vi "format_frame.vi"(6 "mask?":bool, 7 "hangup status code":T1 items=["ignore"=0, "normal"=1000, "going away"=1001, "protocol error"=1002, "invalid data"=1003], 9 "fin?":bool, 10 "data in":string, 11 "opcode":T2 items=["continue"=0, "text"=1, "binary"=2, "hangup"=8, "ping"=9, "pong"=10]) -> (3 "frame data out":string)   [LabVIEW 2019, in "WebSocket Server Toolkit.lvlib"]
uses:
  WebSocket Server Toolkit.lvlib
  types/opcode.ctl
  types/status_code.ctl
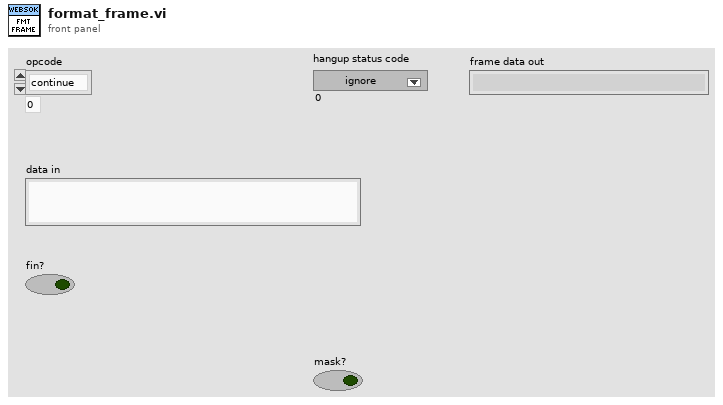
[diagram p1: front panel]
types:
  T1 = typedef "WebSocket Server Toolkit.lvlib/status_code.ctl" = u16
  T2 = typedef "WebSocket Server Toolkit.lvlib/opcode.ctl" = u8
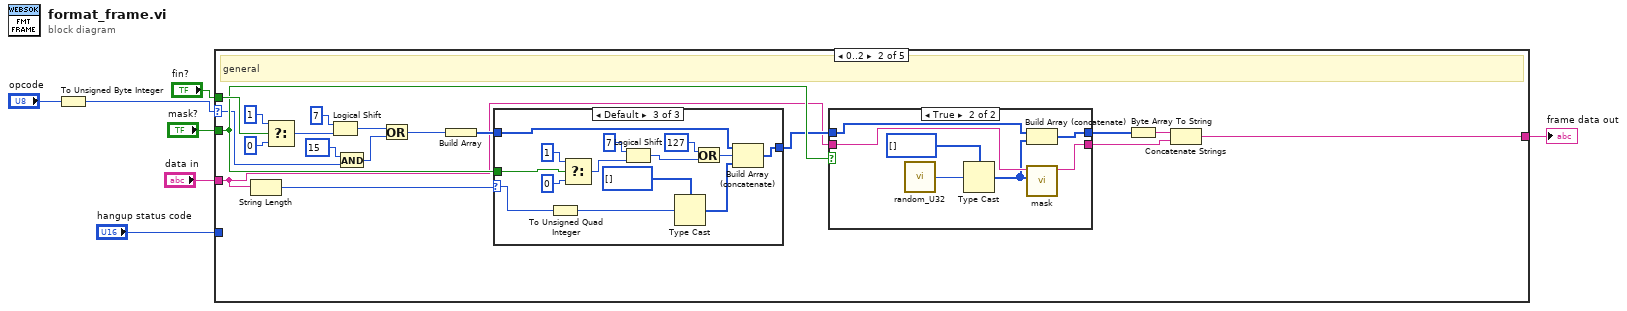
[diagram p0: block diagram]
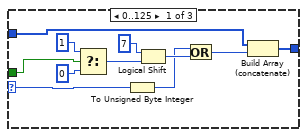
[diagram p4: hidden frame]
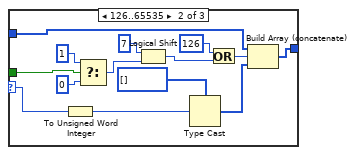
[diagram p5: hidden frame]
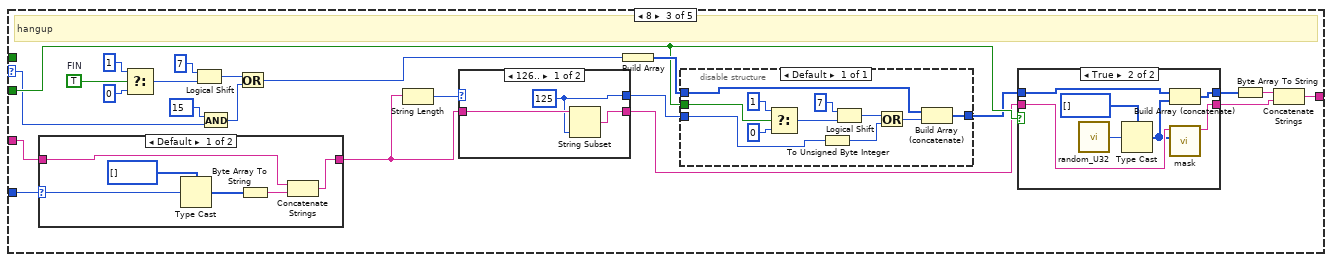
[diagram p6: hidden frame]
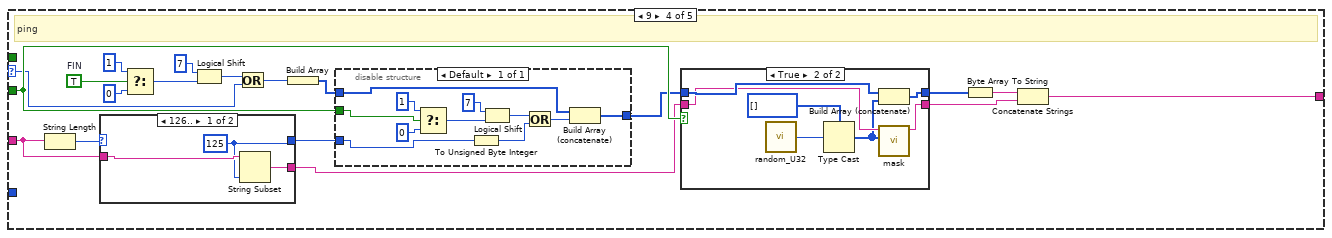
[diagram p10: hidden frame]
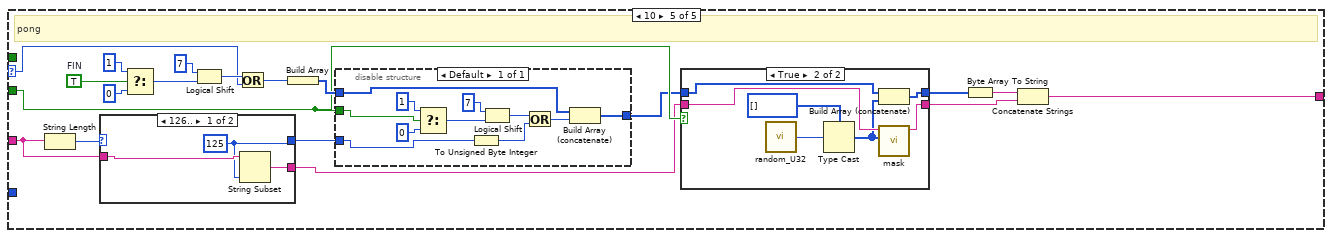
[diagram p13: hidden frame]
diagram:
  n1 = To Unsigned Byte Integer(number="opcode") -> (unsigned 8bit integer=w3:T2)
  n2 = case shown="0..2" w3 {
    selector: w3 -> [_ w10 w76 w130 w174]
    tunnel: "fin?" -> [_ w26 _ _ _]
    tunnel: "data in" -> [_ w15 w84 w134 w178]
    tunnel: "mask?" -> [_ w21 w93 w143 w187]
    tunnel: [_ w17 w89 w139 w183] -> w2
    tunnel: "hangup status code" -> [_ _ w85 _ _]
    frame Default {
    }
    frame 0..2 {
      # "general"
      n3 = String Length(string=w15) -> (length=w14:i32)
      n4 = Select(t=u8 1, s=w26, f=u8 0) -> (s? t:f=w13:u8)
      n5 = Logical Shift(y=i16 7, x=w13) -> (x << y=w8:u8)
      n6 = And(x=i16 15 ("y"), y=w10) -> (x .and. y?=w9:i16)
      n7 = Or(x=w8, y=w9) -> (x .or. y?=w23:i16)
      n8 = Build Array(w23) -> (w22:i16[])
      n9 = case shown="Default" w14 {
        selector: w14 -> [w43 w54 w68]
        tunnel: w21 -> [w44 w58 w72]
        tunnel: w22 -> [w42 w57 w71]
        tunnel: [w40 w55 w69] -> w20
        frame 0..125 {
          n10 = Select(t=u8 1, s=w44, f=u8 0) -> (s? t:f=w38:u8)
          n11 = To Unsigned Byte Integer(number=w43) -> (unsigned 8bit integer=w36:u8)
          n12 = Logical Shift(y=i16 7, x=w38) -> (x << y=w37:u8)
          n13 = Or(x=w36, y=w37) -> (x .or. y?=w41:u8)
          n14 = Build Array (concatenate)(w42, w41) -> (w40:i16[])
        }
        frame 126..65535 {
          n15 = To Unsigned Word Integer(number=w54) -> (unsigned 16bit integer=w53:u16)
          n16 = Select(t=u8 1, s=w58, f=u8 0) -> (s? t:f=w49:u8)
          n17 = Logical Shift(y=i16 7, x=w49) -> (x << y=w48:u8)
          n18 = Type Cast(type=u8[] [], x=w53) -> (*(type *) &x=w51:u8[])
          n19 = Or(x=u8 126, y=w48) -> (x .or. y?=w56:u8)
          n20 = Build Array (concatenate)(w57, w56, w51) -> (w55:i16[])
        }
        frame Default {
          n21 = To Unsigned Quad Integer(1:w68) -> (0:w67:u64)
          n22 = Select(t=u8 1, s=w72, f=u8 0) -> (s? t:f=w63:u8)
          n23 = Logical Shift(y=i16 7, x=w63) -> (x << y=w62:u8)
          n24 = Type Cast(type=u8[] [], x=w67) -> (*(type *) &x=w65:u8[])
          n25 = Or(x=u8 127, y=w62) -> (x .or. y?=w70:u8)
          n26 = Build Array (concatenate)(w71, w70, w65) -> (w69:i16[])
        }
      }
      n27 = case shown="True" w21 {
        tunnel: w20 -> [w28 w33]
        tunnel: [w28 w32] -> w19
        tunnel: [w27 w30] -> w16
        tunnel: w15 -> [w27 w31]
        frame False {
        }
        frame True {
          n28 = call "random_U32.vi"() -> ("random"=w34:u32)  [unwired: 1 in]
          n29 = Type Cast(type=u8[] [], x=w34) -> (*(type *) &x=w29:u8[])
          n30 = Build Array (concatenate)(w33, w29) -> (w32:i16[])
          n31 = call "mask.vi"("mask"=w29, "data in"=w31) -> ("masked data"=w30:string)  [unwired: 9 in]
        }
      }
      n32 = Byte Array To String(unsigned byte array=w19) -> (string=w18:string)
      n33 = Concatenate Strings(w18, w16) -> (w17:string)
    }
    frame 8 {
      w87 = TRUE  # FIN
      # "hangup"
      n34 = case shown="Default" w85 {
        selector: w85 -> [w102 _]
        tunnel: w84 -> [w99 w104]
        tunnel: [w98 w104] -> w82
        frame Default {
          n35 = Type Cast(type=u8[] [], x=w102) -> (*(type *) &x=w101:u8[])
          n36 = Byte Array To String(unsigned byte array=w101) -> (string=w100:string)
          n37 = Concatenate Strings(w99, w100) -> (w98:string)
        }
        frame 0 {
        }
      }
      n38 = Select(t=u8 1, s=w87, f=u8 0) -> (s? t:f=w80:u8)
      n39 = Logical Shift(y=i16 7, x=w80) -> (x << y=w78:u8)
      n40 = And(x=i16 15 ("y"), y=w76) -> (x .and. y?=w75:i16)
      n41 = Or(x=w78, y=w75) -> (x .or. y?=w95:i16)
      n42 = String Length(string=w82) -> (length=w81:i32)
      n43 = case shown="126.." w81 {
        selector: w81 -> [_ w120]
        tunnel: w82 -> [w118 w119]
        tunnel: [w117 w120] -> w86
        tunnel: [w116 w119] -> w83
        frame 126.. {
          w117 = 125 ("length (rest)")
          n44 = String Subset(string=w118, length (rest)=w117) -> (substring=w116:string)  [unwired: 1 in]
        }
        frame Default {
        }
      }
      n45 = Build Array(w95) -> (w94:i16[])
      n46 = disable-structure shown="Default" {
        disable-tunnel: w94 -> [w115]
        disable-tunnel: w93 -> [w114]
        disable-tunnel: [w113] -> w92
        disable-tunnel: w86 -> [w112]
        frame Enabled {
          n47 = Select(t=u8 1, s=w114, f=u8 0) -> (s? t:f=w106:u8)
          n48 = To Unsigned Byte Integer(number=w112) -> (unsigned 8bit integer=w105:u8)
          n49 = Logical Shift(y=i16 7, x=w106) -> (x << y=w108:u8)
          n50 = Or(x=w108, y=w105) -> (x .or. y?=w107:u8)
          n51 = Build Array (concatenate)(w115, w107) -> (w113:i16[])
        }
      }
      n52 = case shown="True" w93 {
        tunnel: w92 -> [w122 w127]
        tunnel: [w122 w126] -> w91
        tunnel: [w121 w124] -> w88
        tunnel: w83 -> [w121 w125]
        frame False {
        }
        frame True {
          n53 = call "random_U32.vi"() -> ("random"=w128:u32)  [unwired: 1 in]
          n54 = Type Cast(type=u8[] [], x=w128) -> (*(type *) &x=w123:u8[])
          n55 = Build Array (concatenate)(w127, w123) -> (w126:i16[])
          n56 = call "mask.vi"("mask"=w123, "data in"=w125) -> ("masked data"=w124:string)  [unwired: 9 in]
        }
      }
      n57 = Byte Array To String(unsigned byte array=w91) -> (string=w90:string)
      n58 = Concatenate Strings(w90, w88) -> (w89:string)
    }
    frame 9 {
      w137 = TRUE  # FIN
      # "ping"
      n59 = String Length(string=w134) -> (length=w133:i32)
      n60 = case shown="126.." w133 {
        selector: w133 -> [_ w164]
        tunnel: w134 -> [w162 w163]
        tunnel: [w161 w164] -> w136
        tunnel: [w160 w163] -> w135
        frame 126.. {
          w161 = 125 ("length (rest)")
          n61 = String Subset(string=w162, length (rest)=w161) -> (substring=w160:string)  [unwired: 1 in]
        }
        frame Default {
        }
      }
      n62 = Select(t=u8 1, s=w137, f=u8 0) -> (s? t:f=w132:u8)
      n63 = Logical Shift(y=i16 7, x=w132) -> (x << y=w131:u8)
      n64 = Or(x=w131, y=w130) -> (x .or. y?=w145:T2)
      n65 = Build Array(w145) -> (w144:T2[])
      n66 = disable-structure shown="Default" {
        disable-tunnel: w144 -> [w159]
        disable-tunnel: w143 -> [w158]
        disable-tunnel: [w157] -> w142
        disable-tunnel: w136 -> [w156]
        frame Enabled {
          n67 = Select(t=u8 1, s=w158, f=u8 0) -> (s? t:f=w151:u8)
          n68 = To Unsigned Byte Integer(number=w156) -> (unsigned 8bit integer=w150:u8)
          n69 = Logical Shift(y=i16 7, x=w151) -> (x << y=w149:u8)
          n70 = Or(x=w149, y=w150) -> (x .or. y?=w152:u8)
          n71 = Build Array (concatenate)(w159, w152) -> (w157:T2[])
        }
      }
      n72 = case shown="True" w143 {
        tunnel: w142 -> [w166 w171]
        tunnel: [w166 w170] -> w141
        tunnel: [w165 w168] -> w138
        tunnel: w135 -> [w165 w169]
        frame False {
        }
        frame True {
          n73 = call "random_U32.vi"() -> ("random"=w172:u32)  [unwired: 1 in]
          n74 = Type Cast(type=u8[] [], x=w172) -> (*(type *) &x=w167:u8[])
          n75 = Build Array (concatenate)(w171, w167) -> (w170:T2[])
          n76 = call "mask.vi"("mask"=w167, "data in"=w169) -> ("masked data"=w168:string)  [unwired: 9 in]
        }
      }
      n77 = Byte Array To String(unsigned byte array=w141) -> (string=w140:string)
      n78 = Concatenate Strings(w140, w138) -> (w139:string)
    }
    frame 10 {
      w181 = TRUE  # FIN
      # "pong"
      n79 = String Length(string=w178) -> (length=w177:i32)
      n80 = case shown="126.." w177 {
        selector: w177 -> [_ w208]
        tunnel: w178 -> [w206 w207]
        tunnel: [w205 w208] -> w180
        tunnel: [w204 w207] -> w179
        frame 126.. {
          w205 = 125 ("length (rest)")
          n81 = String Subset(string=w206, length (rest)=w205) -> (substring=w204:string)  [unwired: 1 in]
        }
        frame Default {
        }
      }
      n82 = Select(t=u8 1, s=w181, f=u8 0) -> (s? t:f=w176:u8)
      n83 = Logical Shift(y=i16 7, x=w176) -> (x << y=w175:u8)
      n84 = Or(x=w175, y=w174) -> (x .or. y?=w189:T2)
      n85 = Build Array(w189) -> (w188:T2[])
      n86 = disable-structure shown="Default" {
        disable-tunnel: w188 -> [w203]
        disable-tunnel: w187 -> [w202]
        disable-tunnel: [w201] -> w186
        disable-tunnel: w180 -> [w200]
        frame Enabled {
          n87 = Select(t=u8 1, s=w202, f=u8 0) -> (s? t:f=w195:u8)
          n88 = To Unsigned Byte Integer(number=w200) -> (unsigned 8bit integer=w193:u8)
          n89 = Logical Shift(y=i16 7, x=w195) -> (x << y=w194:u8)
          n90 = Or(x=w194, y=w193) -> (x .or. y?=w196:u8)
          n91 = Build Array (concatenate)(w203, w196) -> (w201:T2[])
        }
      }
      n92 = case shown="True" w187 {
        tunnel: w186 -> [w210 w215]
        tunnel: [w210 w214] -> w185
        tunnel: [w209 w212] -> w182
        tunnel: w179 -> [w209 w213]
        frame False {
        }
        frame True {
          n93 = call "random_U32.vi"() -> ("random"=w216:u32)  [unwired: 1 in]
          n94 = Type Cast(type=u8[] [], x=w216) -> (*(type *) &x=w211:u8[])
          n95 = Build Array (concatenate)(w215, w211) -> (w214:T2[])
          n96 = call "mask.vi"("mask"=w211, "data in"=w213) -> ("masked data"=w212:string)  [unwired: 9 in]
        }
      }
      n97 = Byte Array To String(unsigned byte array=w185) -> (string=w184:string)
      n98 = Concatenate Strings(w184, w182) -> (w183:string)
    }
  }
  "frame data out" <- w2
